vi "cams.vi"() -> ()   [LabVIEW 2017]
uses:
  <vilib>/userdefined/High Color/IMAQdx.ctl
  <resource>/objmgr/imaqdx.rc
panel:
  in  "Fill in":bool
  in  "OK Button":bool
  in  "CamsToken":string caption="File name"
  in  "CamsDirectory":path caption="Directory"
  out "error out":errorcluster
  in  "Stop":bool
  in  "Camera":T1="Field"
  in  "Launch":bool
  in  "Stop and close":bool
  # "Launcher"
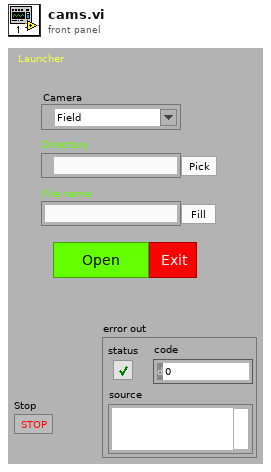
[diagram p1: front panel]
types:
  T1 = typedef "IMAQdx.ctl" = refnum<k21>
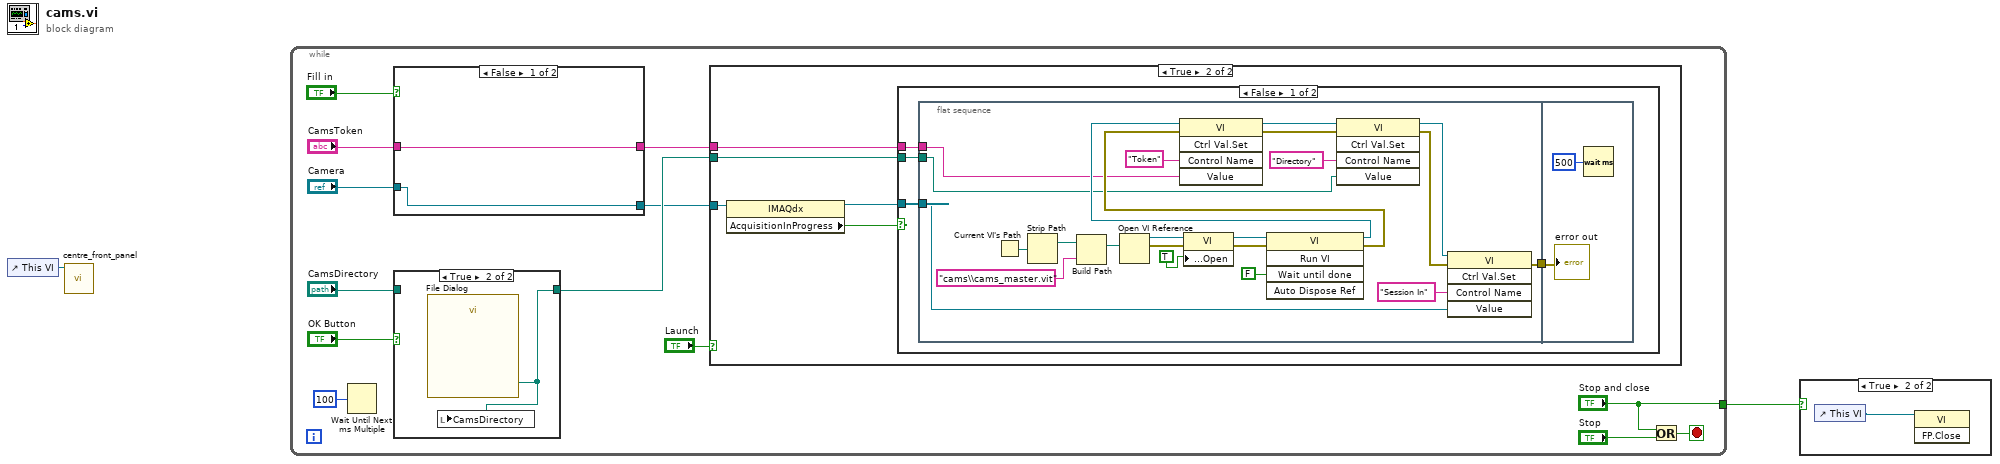
[diagram p0: block diagram]
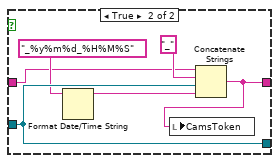
[diagram p3: hidden frame]
diagram:
  n1 = control-ref of="This VI"() -> (w1:refnum<vi>)
  n2 = call "centre_front_panel.vi"("VI in"=w1) -> ()  [unwired: 11 in]
  n3 = while {
    tunnel: ["Stop and close"] -> w2
    stop <- w13 stop-if-true
    n4 = Wait Until Next ms Multiple(millisecond multiple=u32 100) -> ()  [unwired: 1 out]
    n5 = case shown="False" "Fill in" {
      tunnel: [w16 w18] -> w3
      tunnel: "CamsToken" -> [w16 w19]
      tunnel: [w17 w22] -> w5
      tunnel: "Camera" -> [w17 w22]
      frame False {
      }
      frame True {
        n6 = Format Date/Time String(time format string (%c)="_%y%m%d_%H%M%S") -> (date/time string=w23:string)  [unwired: 2 out]
        n7 = Concatenate Strings(w19, "_" ("string"), w22, w23) -> (w18:string)
        n8 = local write "CamsToken"(w18) -> ()
      }
    }
    n9 = case shown="True" "OK Button" {
      tunnel: [w24 w25] -> w8
      tunnel: "CamsDirectory" -> [w24 _]
      frame False {
      }
      frame True {
        n10 = call "File Dialog"() -> ("selected path"=w25:path)  [unwired: 12 in, 3 out]
        n11 = local write "CamsDirectory"(w25) -> ()
      }
    }
    n12 = case shown="True" "Launch" {
      tunnel: w8 -> [_ w28]
      tunnel: w5 -> [_ w27]
      tunnel: w3 -> [_ w26]
      frame False {
      }
      frame True {
        n13 = property class="IMAQdx"(reference=w27) -> (reference out=w29:T1, "AcquisitionInProgress"=w30:bool)  [unwired: 1 in, 1 out]
        n14 = case shown="False" w30 {
          tunnel: w29 -> [w34 _]
          tunnel: w28 -> [w32 _]
          tunnel: w26 -> [w31 _]
          frame False {
            n15 = flat-sequence {
              tunnel: w34 -> [w45]
              tunnel: [w57] -> w33
              tunnel: w32 -> [w36]
              tunnel: w31 -> [w35]
              tunnel: w33 -> [w58]
              frame #0 {
                n16 = Current VI's Path() -> (path=w53:path)
                n17 = Strip Path(path=w53) -> (stripped path=w54:path)  [unwired: 1 out]
                n18 = Build Path(base path=w54, name or relative path="cams\\cams_master.vit") -> (appended path=w55:path)
                n19 = Open VI Reference(vi path=w55) -> (vi reference=w49:refnum<vi>, error out=w51:errorcluster)  [unwired: 5 in]
                n20 = property on="Property Node" class="VI"(reference=w49, error in=w51, "Front Panel Window:Open"=TRUE) -> (reference out=w50:refnum<vi>, error out=w52:errorcluster)
                n21 = invoke class="VI" method="Run VI"(reference=w50, error in=w52, "Wait until done"=FALSE) -> (reference out=w44:refnum<vi>, error out=w43:errorcluster)  [unwired: 2 in, 3 out]
                n22 = invoke class="VI" method="Ctrl Val.Set"(reference=w44, error in=w43, "Control Name"="Token", "Value"=w35) -> (reference out=w42:refnum<vi>, error out=w41:errorcluster)  [unwired: 1 in, 3 out]
                n23 = invoke class="VI" method="Ctrl Val.Set"(reference=w42, error in=w41, "Control Name"="Directory", "Value"=w36) -> (reference out=w40:refnum<vi>, error out=w39:errorcluster)  [unwired: 1 in, 3 out]
                n24 = invoke class="VI" method="Ctrl Val.Set"(reference=w40, error in=w39, "Control Name"="Session In", "Value"=w45) -> (error out=w57:errorcluster)  [unwired: 1 in, 4 out]
              }
              frame #1 {
                n25 = Wait (ms)(milliseconds to wait=u32 500) -> ()  [unwired: 1 out]
                "error out" <- w58
              }
            }
          }
          frame True {
          }
        }
      }
    }
    n26 = Or(x="Stop and close", y="Stop") -> (x .or. y?=w13:bool)
  }
  n27 = case shown="True" w2 {
    frame False {
    }
    frame True {
      n28 = control-ref of="This VI"() -> (w60:refnum<vi>)
      n29 = invoke class="VI" method="FP.Close"(reference=w60) -> ()  [unwired: 2 in, 3 out]
    }
  }
